vi "RDS Serial Handle Frame.vi"(8 "error in (no error)":errorcluster, 10 "RDS Serial Frame":refnum<class "RDS Serial Frame.lvclass">, 11 "AIP Instrument in":refnum<class "AIP Instrument.lvclass">) -> (0 "error out":errorcluster, 3 "AIP Instrument out":refnum<class "AIP Instrument.lvclass">)   [LabVIEW 2015, in "AIP Instrument.lvlib" / "AIP Instrument.lvclass"]
uses:
  AIP Instrument.lvclass
  Libraries/RDS Serial Handler/RDS Serial Frame.lvclass
  Actors/RDS Parent Actor/RDS Parent Actor/RDS Parent Actor.lvclass
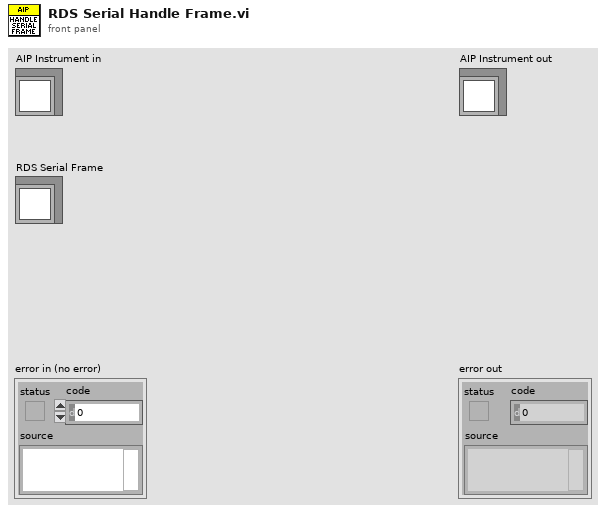
[diagram p1: front panel]
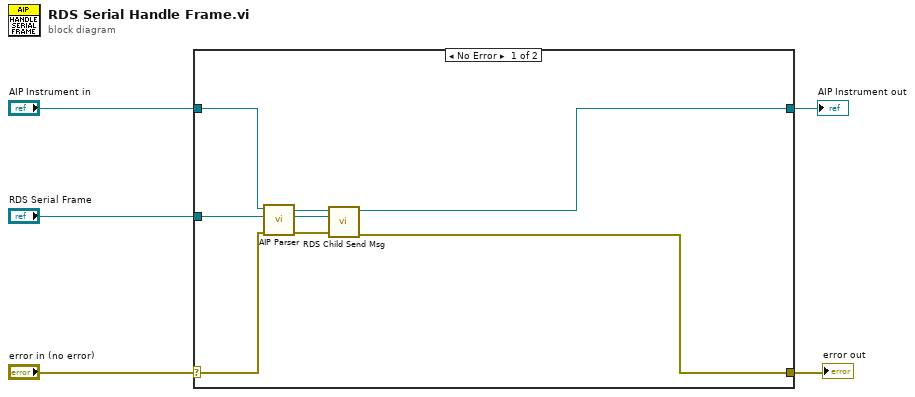
[diagram p0: block diagram]
diagram:
  n1 = case shown="No Error" "error in (no error)" {
    selector: "error in (no error)" -> [w7 w15]
    tunnel: [w6 w15] -> w2
    tunnel: [w8 w14] -> w1
    tunnel: "AIP Instrument in" -> [w13 w14]
    tunnel: "RDS Serial Frame" -> [w12 _]
    frame No Error {
      n2 = call "AIP Parser.vi"("error in (no error)"=w7, "RDS Serial Frame"=w12, "AIP Instrument in"=w13) -> ("error out"=w9:errorcluster, "AIP Status Response"=w10:refnum<class "AIP Status Response.lvclass">, "AIP Instrument out"=w11:refnum<class "AIP Instrument.lvclass">)  [unwired: 6 in]
      n3 = call "RDS Child Send Msg.vi"("error in (no error)"=w9, "RDS Message"=w10, "RDS Parent Actor in"=w11) -> ("error out"=w6:errorcluster, "RDS Parent Actor out"=w8:refnum<class "AIP Instrument.lvclass">)  [unwired: 7 in]
    }
    frame Error {
    }
  }
  "error out" <- w2
  "AIP Instrument out" <- w1
